vi "driveCodeArcade.vi"(6 "maxSpeed":dbl, 8 "joystick":T5={"Device"=enum."USB 1"}, 10 "rightMotor":T1={"DeviceStatus"={"status"=FALSE, "code"=0, "source"=""}, "Type"=enum."PWM", "PWM"={"PWM Channel"=enum."PWM 1", "DeadBand"={"Name"="", "maxPositivePwm"=0, "minPositivePwm"=0, "centerPwm"=0, "maxNegativePwm"=0, "minNegativePwm"=0, "angularRange"=0}}, "CAN"={"Device Number"=0, "SetOutput VI Ref"=variant(enum8{"Percent VBus", "Current", "Speed", "Position", "Voltage"} enum."Percent VBus"), "GetOutput VI Ref"=variant(refnum<k1> refnum), "Enable VI Ref"=variant(dbl 12.0), "Disable VI Ref"=variant(enum8{"Percent VBus", "Speed", "Position", "Slave", "Unchanged / Invalid", "Voltage Compensation", "Current", "Motion Profile"} enum."Percent VBus"), "Data"=variant}, "Invert"=FALSE}, 11 "leftMotor":T1={"DeviceStatus"={"status"=FALSE, "code"=0, "source"=""}, "Type"=enum."PWM", "PWM"={"PWM Channel"=enum."PWM 1", "DeadBand"={"Name"="", "maxPositivePwm"=0, "minPositivePwm"=0, "centerPwm"=0, "maxNegativePwm"=0, "minNegativePwm"=0, "angularRange"=0}}, "CAN"={"Device Number"=0, "SetOutput VI Ref"=variant(enum8{"Percent VBus", "Current", "Speed", "Position", "Voltage"} enum."Percent VBus"), "GetOutput VI Ref"=variant(refnum<k1> refnum), "Enable VI Ref"=variant(dbl 12.0), "Disable VI Ref"=variant(enum8{"Percent VBus", "Speed", "Position", "Slave", "Unchanged / Invalid", "Voltage Compensation", "Current", "Motion Profile"} enum."Percent VBus"), "Data"=variant}, "Invert"=FALSE}) -> (0 "rightSpeed":dbl, 1 "leftSpeed":dbl, 2 "rightMotor":T1={"DeviceStatus"={"status"=FALSE, "code"=0, "source"=""}, "Type"=enum."PWM", "PWM"={"PWM Channel"=enum."PWM 1", "DeadBand"={"Name"="", "maxPositivePwm"=0, "minPositivePwm"=0, "centerPwm"=0, "maxNegativePwm"=0, "minNegativePwm"=0, "angularRange"=0}}, "CAN"={"Device Number"=0, "SetOutput VI Ref"=variant(enum8{"Percent VBus", "Current", "Speed", "Position", "Voltage"} enum."Percent VBus"), "GetOutput VI Ref"=variant(refnum<k1> refnum), "Enable VI Ref"=variant(dbl 12.0), "Disable VI Ref"=variant(enum8{"Percent VBus", "Speed", "Position", "Slave", "Unchanged / Invalid", "Voltage Compensation", "Current", "Motion Profile"} enum."Percent VBus"), "Data"=variant}, "Invert"=FALSE}, 3 "leftMotor":T1={"DeviceStatus"={"status"=FALSE, "code"=0, "source"=""}, "Type"=enum."PWM", "PWM"={"PWM Channel"=enum."PWM 1", "DeadBand"={"Name"="", "maxPositivePwm"=0, "minPositivePwm"=0, "centerPwm"=0, "maxNegativePwm"=0, "minNegativePwm"=0, "angularRange"=0}}, "CAN"={"Device Number"=0, "SetOutput VI Ref"=variant(enum8{"Percent VBus", "Current", "Speed", "Position", "Voltage"} enum."Percent VBus"), "GetOutput VI Ref"=variant(refnum<k1> refnum), "Enable VI Ref"=variant(dbl 12.0), "Disable VI Ref"=variant(enum8{"Percent VBus", "Speed", "Position", "Slave", "Unchanged / Invalid", "Voltage Compensation", "Current", "Motion Profile"} enum."Percent VBus"), "Data"=variant}, "Invert"=FALSE})   [LabVIEW 2016]
uses:
  <vilib>/Rock Robotics/WPI/MotorControl/WPI_MotorControlDeviceRef.ctl
  <vilib>/Rock Robotics/WPI/MotorControl/WPI_MotorControlType.ctl
  <vilib>/Rock Robotics/SystemInterfaces/DIO/FPGA_DIOPWMChannel.ctl
  <vilib>/Rock Robotics/WPI/PWM/WPI_PWMDeadband.ctl
  <vilib>/Rock Robotics/WPI/Joystick/WPI_JoystickDevRef.ctl
  <vilib>/Rock Robotics/WPI/Joystick/WPI_JoystickDeviceEnum.ctl
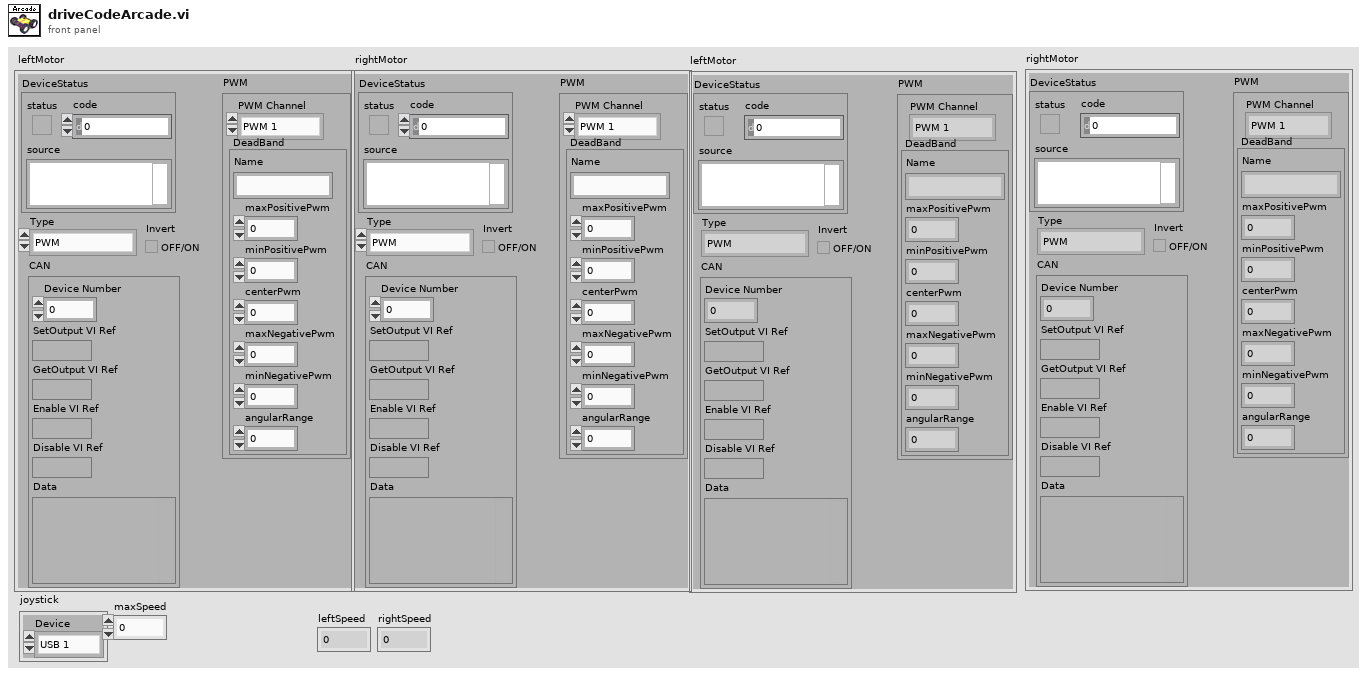
[diagram p1: front panel]
types:
  T1 = typedef "WPI_MotorControlDeviceRef.ctl" = cluster{"DeviceStatus":errorcluster, "Type":T2, "PWM":cluster{"PWM Channel":T3, "DeadBand":T4}, "CAN":cluster{"Device Number":u8, "SetOutput VI Ref":variant, "GetOutput VI Ref":variant, "Enable VI Ref":variant, "Disable VI Ref":variant, "Data":variant}, "Invert":bool}
  T2 = typedef "WPI_MotorControlType.ctl" = enum16{"PWM", "CAN"}
  T3 = typedef "FPGA_DIOPWMChannel.ctl" = enum8{"PWM 0", "PWM 1", "PWM 2", "PWM 3", "PWM 4", "PWM 5", "PWM 6", "PWM 7", "PWM 8", "PWM 9", "PWM MXP 0", "PWM MXP 1", "PWM MXP 2", "PWM MXP 3", "PWM MXP 4", "PWM MXP 5", "PWM MXP 6", "PWM MXP 7", "PWM MXP 8", "PWM MXP 9", "Invalid"}
  T4 = typedef "WPI_PWMDeadband.ctl" = cluster{"Name":string, "maxPositivePwm":i32, "minPositivePwm":i32, "centerPwm":i32, "maxNegativePwm":i32, "minNegativePwm":i32, "angularRange":u16}
  T5 = typedef "WPI_JoystickDevRef.ctl" = cluster{"Device":T6}
  T6 = typedef "WPI_JoystickDeviceEnum.ctl" = enum16{"USB 0", "USB 1", "USB 2", "USB 3", "USB 4", "USB 5"}
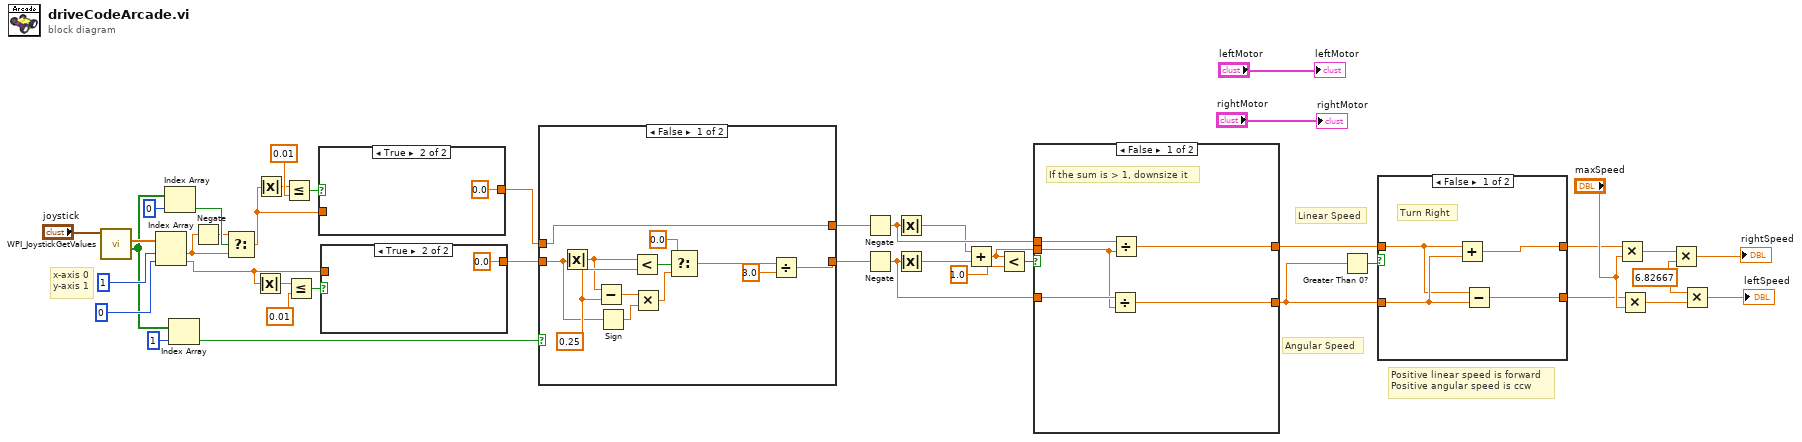
[diagram p0: block diagram]
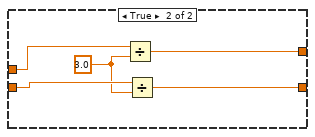
[diagram p4: hidden frame]
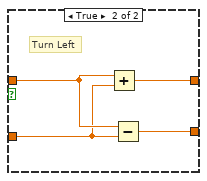
[diagram p5: hidden frame]
diagram:
  w20 = 6.82667 ("y")
  # "Angular Speed"
  # "Positive linear speed is forward\nPositive angular speed is ccw"
  # "Linear Speed"
  # "x-axis 0\ny-axis 1"
  n1 = call <vilib>:"WPI_JoystickGetValues.vi"("JoystickDevRef"="joystick") -> ("Buttons"=w15:bool[], "Axes"=w42:dbl[])  [unwired: 6 in, 3 out]
  n2 = Index Array(array=w42, index #1=1 ("index"), index #2=0 ("index")) -> (element #1=w16:dbl, element #2=w3:dbl)
  n3 = Index Array(array=w15, index=0) -> (element=w18:bool)
  n4 = Index Array(array=w15, index=1) -> (element=w13:bool)
  n5 = Negate(x=w16) -> (-x=w17:dbl)
  n6 = Select(t=w17, s=w18, f=w16) -> (s? t:f=w1:dbl)
  n7 = Absolute Value(x=w3) -> (abs(x)=w4:dbl)
  n8 = Absolute Value(x=w1) -> (abs(x)=w2:dbl)
  n9 = Less Or Equal?(x=w2, y=0.01) -> (x <= y?=w10:bool)
  n10 = Less Or Equal?(x=w4, y=0.01) -> (x <= y?=w9:bool)
  n11 = case shown="True" w10 {
    tunnel: [w44 0.0 ("upper limit")] -> w8
    tunnel: w1 -> [w44 _]
    frame False {
    }
    frame True {
    }
  }
  n12 = case shown="True" w9 {
    tunnel: [w46 0.0 ("upper limit")] -> w7
    tunnel: w3 -> [w46 _]
    frame False {
    }
    frame True {
    }
  }
  n13 = case shown="False" w13 {
    tunnel: [w59 w64] -> w12
    tunnel: [w50 w63] -> w11
    tunnel: w7 -> [w51 w62]
    tunnel: w8 -> [w59 w61]
    frame False {
      w56 = 0.25 ("y")
      n14 = Absolute Value(x=w51) -> (abs(x)=w55:dbl)
      n15 = Subtract(x=w55, y=w56) -> (x-y=w54:dbl)
      n16 = Sign(1:w51) -> (0:w52:dbl)
      n17 = Less?(x=w55, y=w56) -> (x < y?=w58:bool)
      n18 = Multiply(x=w54, y=w52) -> (x*y=w53:dbl)
      n19 = Select(t=0.0, s=w58, f=w53) -> (s? t:f=w49:dbl)
      n20 = Divide(x=w49, y=3.0) -> (x/y=w50:dbl)
    }
    frame True {
      w60 = 3.0 ("y")
      n21 = Divide(x=w61, y=w60) -> (x/y=w64:dbl)
      n22 = Divide(x=w62, y=w60) -> (x/y=w63:dbl)
    }
  }
  n23 = Negate(x=w12) -> (-x=w35:dbl)
  n24 = Negate(x=w11) -> (-x=w32:dbl)
  n25 = Absolute Value(x=w35) -> (abs(x)=w34:dbl)
  n26 = Absolute Value(x=w32) -> (abs(x)=w33:dbl)
  n27 = Add(x=w34, y=w33) -> (x+y=w31:dbl)
  n28 = Less?(x=w31, y=1.0) -> (x < y?=w38:bool)
  n29 = case shown="False" w38 {
    tunnel: w35 -> [w69 w71]
    tunnel: w32 -> [w68 w70]
    tunnel: [w67 w71] -> w28
    tunnel: [w66 w70] -> w26
    tunnel: w31 -> [w65 _]
    frame False {
      # "If the sum is > 1, downsize it"
      n30 = Divide(x=w68, y=w65) -> (x/y=w66:dbl)
      n31 = Divide(x=w69, y=w65) -> (x/y=w67:dbl)
    }
    frame True {
      # "If the sum of angular and linear velocity\nis < 1, keep the joystick values"
    }
  }
  n32 = Greater Than 0?(x=w26) -> (x > 0?=w29:bool)
  n33 = case shown="False" w29 {
    tunnel: w26 -> [w74 w76]
    tunnel: w28 -> [w73 w77]
    tunnel: [w75 w79] -> w27
    tunnel: [w72 w78] -> w25
    frame False {
      # "Turn Right"
      n34 = Add(x=w73, y=w74) -> (x+y=w75:dbl)
      n35 = Subtract(x=w73, y=w74) -> (x-y=w72:dbl)
    }
    frame True {
      # "Turn Left"
      n36 = Add(x=w77, y=w76) -> (x+y=w79:dbl)
      n37 = Subtract(x=w77, y=w76) -> (x-y=w78:dbl)
    }
  }
  n38 = Multiply(x=w27, y="maxSpeed") -> (x*y=w24:dbl)
  n39 = Multiply(x=w25, y="maxSpeed") -> (x*y=w22:dbl)
  n40 = Multiply(x=w24, y=w20) -> (x*y=→"rightSpeed":dbl)
  n41 = Multiply(x=w20, y=w22) -> (x*y=→"leftSpeed":dbl)
  "leftMotor" <- "leftMotor"
  "rightMotor" <- "rightMotor"
